vi "Get Date String.vi"(8 "Display State In":cluster{"Month":i32, "Day":i32, "Year":i32}={"Month"=8, "Day"=1, "Year"=2022}) -> (0 "Date String Out":string)   [LabVIEW 2019, in "Custom Calendar.xctl"]
uses:
  Custom Calendar.xctl
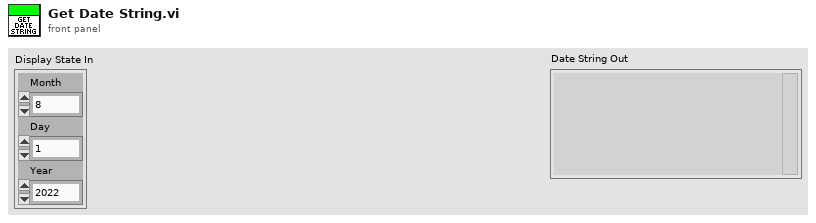
[diagram p1: front panel]
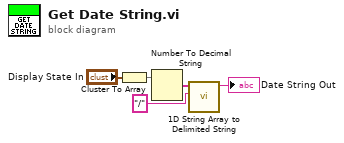
[diagram p0: block diagram]
diagram:
  n1 = Cluster To Array(cluster="Display State In") -> (array=w4:i32[])
  n2 = Number To Decimal String(number=w4) -> (decimal integer string=w5:string[])  [unwired: 1 in]
  n3 = call <vilib>:"1D String Array to Delimited String.vi"("delimiter"="/", "string array"=w5) -> ("delimited string"=→"Date String Out":string)  [unwired: 9 in]
